vi "trend.vi"() -> ()   [LabVIEW 2014]
panel:
  in  "Turns":i64
  in  "Penalty":dbl
  in  "Life Points":i64
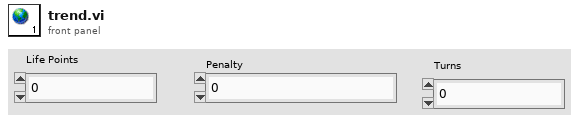
[diagram p1: front panel]
diagram:
